vi "ListeningTask.vi"(8 "error in (no error)":errorcluster) -> (0 "error out":errorcluster)   [LabVIEW 2014, in "UmlEditor.lvclass"]
uses:
  <resource>/Framework/Providers/Open_GDS/UML/UmlEditor_class/UmlEditor.lvclass
  <resource>/Framework/Providers/Open_GDS/UML/UmlEditor_class/EventData.ctl
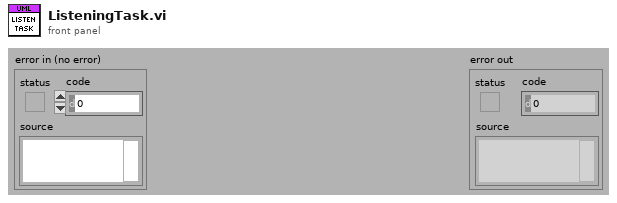
[diagram p1: front panel]
types:
  T1 = typedef "UmlEditor.lvclass/EventData.ctl" = cluster{"Action":string, "Data":string}
  T2 = cluster{"Counter":i32, "Text":string, "Cancelled":bool}
  T3 = typedef "UmlEditor.lvclass/ObjectAttributes.ctl" = cluster{"ListeningQueueIn":refnum<queue>, "Event":refnum<user-event>, "UseProjectFolderAsBasePath":bool, "TypeSyncOption":bool, "Attr":string[], "ToolTip":cluster{"ToolTipOpen":bool, "LastToolTip":i32}, "ClassesToIgnore":string[], "UndoSize":i32, "OpenLastSavedFileWhenStarting":bool, "SyncOption":T4, "SyncTime(s)":i32, "Params":cluster{"IniParams":T5, "Value":string}[], "GraphButtons":refnum<vi>}
  T4 = typedef "UMLEditor_SyncOptions.ctl" = cluster{"IgnoreInstrLib":bool, "IgnoreUserLib":bool, "IgnoreViLib":bool}
  T5 = typedef "UmlEditor.lvclass/IniParamsType.ctl" = enum16{"I have problem with UML stability on my computer"}
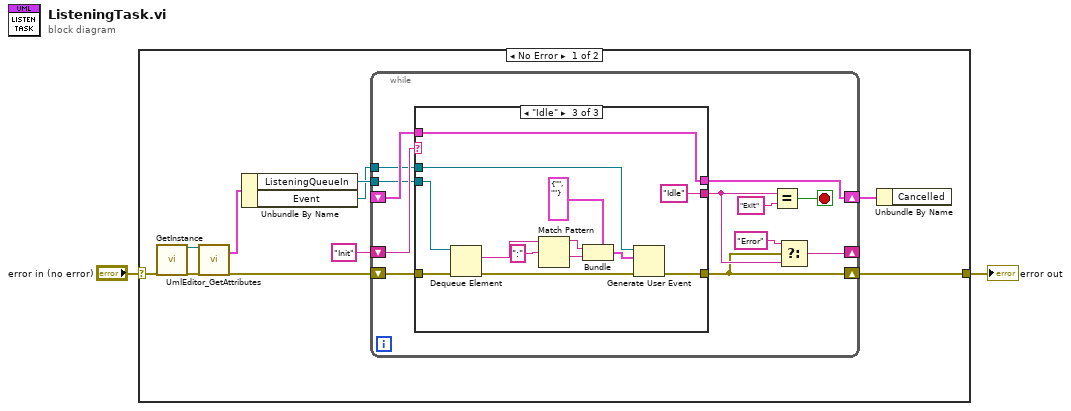
[diagram p0: block diagram]
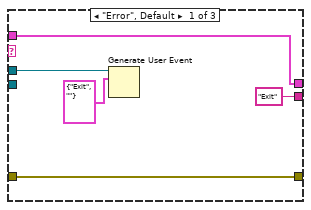
[diagram p2: hidden frame]
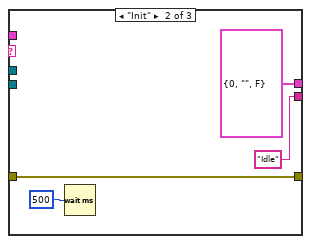
[diagram p3: hidden frame]
diagram:
  n1 = case shown="No Error" "error in (no error)" {
    selector: "error in (no error)" -> [w10 w47]
    tunnel: [w6 w47] -> w1
    frame No Error {
      n2 = call <resource>:"GetInstance.vi"("error in (no error)"=w10) -> ("reference out"=w11:refnum<class "UmlEditor.lvclass">, "error out"=w12:errorcluster)  [unwired: 17 out]
      n3 = call <resource>:"UmlEditor_GetAttributes.vi"("reference in"=w11, "error in (no error)"=w12) -> ("Data"=w3:T3, "error out"=w7:errorcluster)  [unwired: 1 in, 15 out]
      n4 = Unbundle By Name(w3) -> ("ListeningQueueIn"=w5:refnum<queue>, "Event"=w4:refnum<user-event>)
      n5 = while {
        shift-right: [w17] -> w6
        shift-left: w7 -> [w24]
        shift-right: [w22] -> _
        shift-left: "Init" -> [w23]
        shift-right: [w16] -> w8
        shift-left: _ -> [w15]
        tunnel: w5 -> [w14]
        tunnel: w4 -> [w13]
        stop <- w21 stop-if-true
        n6 = case shown="\"Idle\"" w23 {
          tunnel: w24 -> [w29 w32 w45]
          tunnel: [w29 w32 w41] -> w17
          tunnel: ["Exit" "Idle" "Idle"] -> w18
          tunnel: [w27 T2 {"Counter"=0, "Text"="", "Cancelled"=FALSE} w35] -> w16
          tunnel: w15 -> [w27 _ w35]
          tunnel: w14 -> [_ _ w44]
          tunnel: w13 -> [w26 _ w40]
          frame "Error", Default {
            n7 = Generate User Event(user event=w26, event data cluster=T1 {"Action"="Exit", "Data"=""} ("event data")) -> ()  [unwired: 2 in, 2 out]
          }
          frame "Init" {
            n8 = Wait (ms)(milliseconds to wait=u32 500) -> ()  [unwired: 1 out]
          }
          frame "Idle" {
            n9 = Dequeue Element(queue=w44, error in (no error)=w45) -> (element=w34:string, error out=w42:errorcluster)  [unwired: 3 out]
            n10 = Match Pattern(string=w34, regular expression=":") -> (before substring=w37:string, after substring=w36:string)  [unwired: 3 out]
            n11 = Bundle(cluster=T1 {"Action"="", "Data"=""} ("event data"), "Action"=w37, "Data"=w36) -> (w38:T1)
            n12 = Generate User Event(user event=w40, event data cluster=w38, error in=w42) -> (error out=w41:errorcluster)  [unwired: 1 in, 1 out]
          }
        }
        n13 = Equal?(x=w18, y="Exit") -> (x = y?=w21:bool)
        n14 = Select(t="Error", s=w17, f=w18) -> (s? t:f=w22:string)
      }
      n15 = Unbundle By Name(w8) -> ()  [unwired: 1 out]
    }
    frame Error {
    }
  }
  "error out" <- w1
